vi "GetControlNames.vi"(8 "error in (no error)":errorcluster, 11 "VI in":refnum<vi>) -> (0 "error out":errorcluster, 2 "Array 2":string[](array[string]), 3 "Array":refnum<vi>[](array[refnum]))   [LabVIEW 2017]
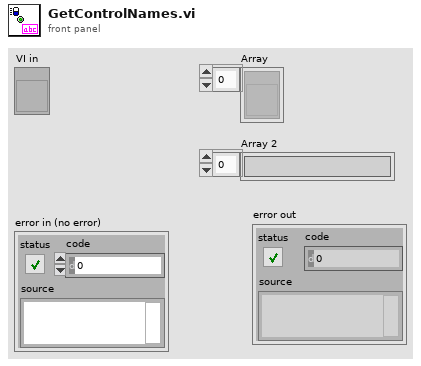
[diagram p1: front panel]
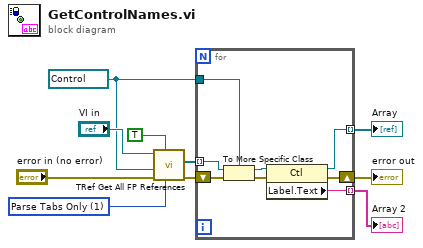
[diagram p0: block diagram]
diagram:
  w4 = u16 1 items=["Parse All", "Parse Tabs Only"] ("Parsing Rule")
  w6 = refnum<vi> refnum ("Ctl Refnum")
  n1 = call <vilib>:"TRef Get All FP References.vi"("Parsing Rule"=w4, "Ignore Decorations?"=TRUE, "error in (no error)"="error in (no error)", "GObj Refnum"=w6, "VI Refnum"="VI in") -> ("error out"=w5:errorcluster, "All FP Objects"=w7:refnum<vi>[])  [unwired: 2 in, 3 out]
  n2 = for {
    shift-right: [w18] -> w1
    shift-left: w5 -> [w15]
    tunnel: [w17] -> w8 mode=indexing
    tunnel: [w16] -> w9 mode=indexing
    tunnel: w6 -> [w13]
    tunnel: w7 -> [w12] mode=indexing
    n3 = To More Specific Class(target class=w13, reference=w12, error in=w15) -> (specific class reference=w11:refnum<vi>, error out=w14:errorcluster)
    n4 = property class="Ctl"(reference=w11, error in=w14) -> (reference out=w16:refnum<vi>, error out=w18:errorcluster, "Label.Text"=w17:string)
  }
  "Array" <- w9
  "Array 2" <- w8
  "error out" <- w1
